vi "Max Bin Read (single queue).vi"(0 "FPGA VI Reference In":refnum<k20>) -> (14 "Max Bin":i32, 15 "Max Amp":dbl, 16 "Next Bin":i32, 17 "Next Amp":dbl, 18 "Prev Bin":i32, 19 "Prev Amp":dbl)   [LabVIEW 2014]
uses:
  <vilib>/Utility/error.llb/Error Cluster From Error Code.vi
  <vilib>/rvi/errors/niLvFpgaAdjustHostInterfaceError.vi
  <vilib>/rvi/interface/nirviMethod/nirviMethod.xnode
  <vilib>/FPGAPlugInAG/Dynamic/niLvFpga_ReadFifo_Dynamic.vi
  <vilib>/rvi/errors/niLvFpgaMergeErrorWithErrorCode.vi
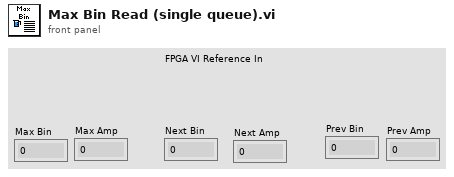
[diagram p1: front panel]
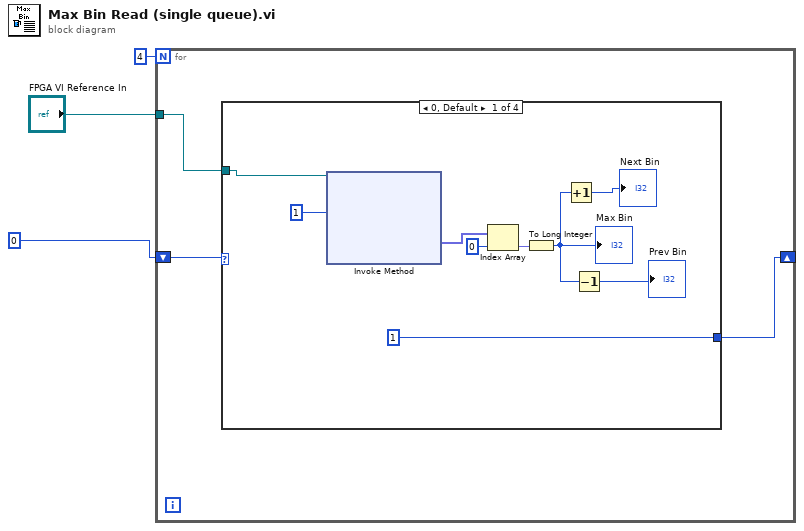
[diagram p0: block diagram]
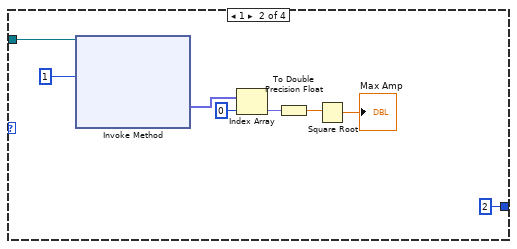
[diagram p2: hidden frame]
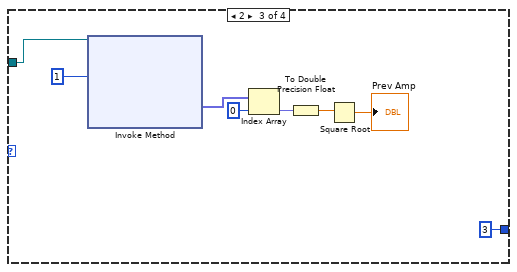
[diagram p3: hidden frame]
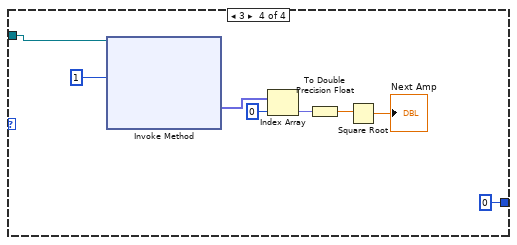
[diagram p4: hidden frame]
diagram:
  n1 = for {
    N: 4 -> [_]
    tunnel: "FPGA VI Reference In" -> [w6]
    shift-right: [w5] -> _
    shift-left: 0 -> [w4]
    n2 = case shown="0, Default" w4 {
      tunnel: w6 -> [w12 w23 w25 w33]
      tunnel: [1 2 3 0] -> w5
      frame 0, Default {
        n3 = xnode "Invoke Method"("FPGA VI Reference In"=w12, "Number of Elements"=u32 1) -> ("Data"=w14:fxp<+,44,44>[])  [unwired: 2 in, 3 out]
        n4 = Index Array(array=w14, index=0) -> (element=w11:fxp<+,44,44>)
        n5 = To Long Integer(number=w11) -> (32bit integer=w10:i32)
        "Max Bin" <- w10
        n6 = Increment(x=w10) -> (x+1=→"Next Bin":i32)
        n7 = Decrement(x=w10) -> (x-1=→"Prev Bin":i32)
      }
      frame 1 {
        n8 = xnode "Invoke Method"("FPGA VI Reference In"=w23, "Number of Elements"=u32 1) -> ("Data"=w21:fxp<+,44,44>[])  [unwired: 2 in, 3 out]
        n9 = Index Array(array=w21, index=0) -> (element=w19:fxp<+,44,44>)
        n10 = To Double Precision Float(number=w19) -> (double precision float=w18:dbl)
        n11 = Square Root(x=w18) -> (sqrt(x)=→"Max Amp":dbl)
      }
      frame 2 {
        n12 = xnode "Invoke Method"("FPGA VI Reference In"=w25, "Number of Elements"=u32 1) -> ("Data"=w30:fxp<+,44,44>[])  [unwired: 2 in, 3 out]
        n13 = Index Array(array=w30, index=0) -> (element=w28:fxp<+,44,44>)
        n14 = To Double Precision Float(number=w28) -> (double precision float=w27:dbl)
        n15 = Square Root(x=w27) -> (sqrt(x)=→"Prev Amp":dbl)
      }
      frame 3 {
        n16 = xnode "Invoke Method"("FPGA VI Reference In"=w33, "Number of Elements"=u32 1) -> ("Data"=w35:fxp<+,44,44>[])  [unwired: 2 in, 3 out]
        n17 = Index Array(array=w35, index=0) -> (element=w37:fxp<+,44,44>)
        n18 = To Double Precision Float(number=w37) -> (double precision float=w38:dbl)
        n19 = Square Root(x=w38) -> (sqrt(x)=→"Next Amp":dbl)
      }
    }
  }
